vi "Get sampling info.vi"(8 "error in (no error)":errorcluster, 11 "Generator in":refnum<class "Generador.lvclass">) -> (0 "error out":errorcluster, 2 "sampling info":cluster{"Fs":dbl, "#s":dbl}={"Fs"=1000.0, "#s"=1000.0} {"Fs" format="%.2p"}, 3 "Generator out":refnum<class "Generador.lvclass">)   [LabVIEW 2020, in "FGen.lvlib" / "Generador.lvclass"]
uses:
  Generador.lvclass
  Generador.lvclass/Generador.ctl
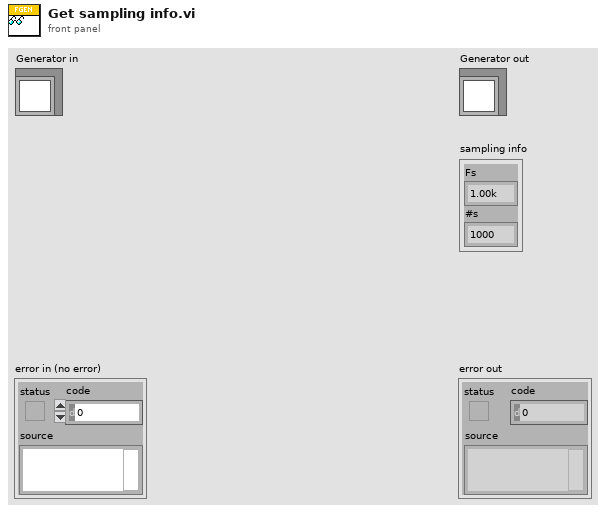
[diagram p1: front panel]
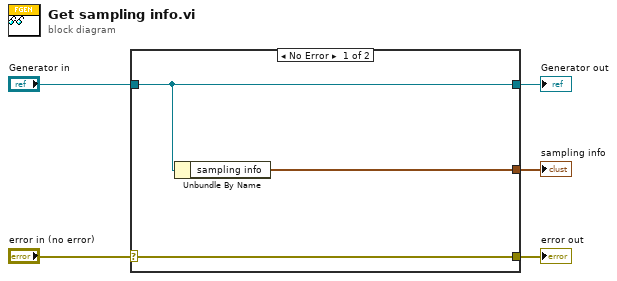
[diagram p0: block diagram]
diagram:
  n1 = case shown="No Error" "error in (no error)" {
    selector: "error in (no error)" -> [w8 w9]
    tunnel: [w8 w9] -> w4
    tunnel: [w7 w10] -> w2
    tunnel: "Generator in" -> [w7 w10]
    tunnel: [w6 _] -> w1
    frame No Error {
      n2 = Unbundle By Name(w7) -> ("sampling info"=w6:cluster{"Fs":dbl, "#s":dbl})
    }
    frame Error {
    }
  }
  "error out" <- w4
  "Generator out" <- w2
  "sampling info" <- w1
